vi "Add Event Reference to maps.vi"(7 "New Node Path":string, 8 "Event type":T1, 9 "Event VIs":refnum<vi>[](array[refnum]), 10 "Tree Map in":T2, 11 "map ref in":map{string, refnum<vi>}(c390)) -> (2 "Tree Map out":T2, 3 "map ref out":map{string, refnum<vi>}(c390))   [LabVIEW 2019, in "Panther Dashboard.lvlib"]
uses:
  Panther Dashboard.lvlib
  <vilib>/National Instruments/Tree Map/Tree Map Data.ctl
  Event types--enum.ctl
  <vilib>/National Instruments/Tree Map/Tree Map.lvlib
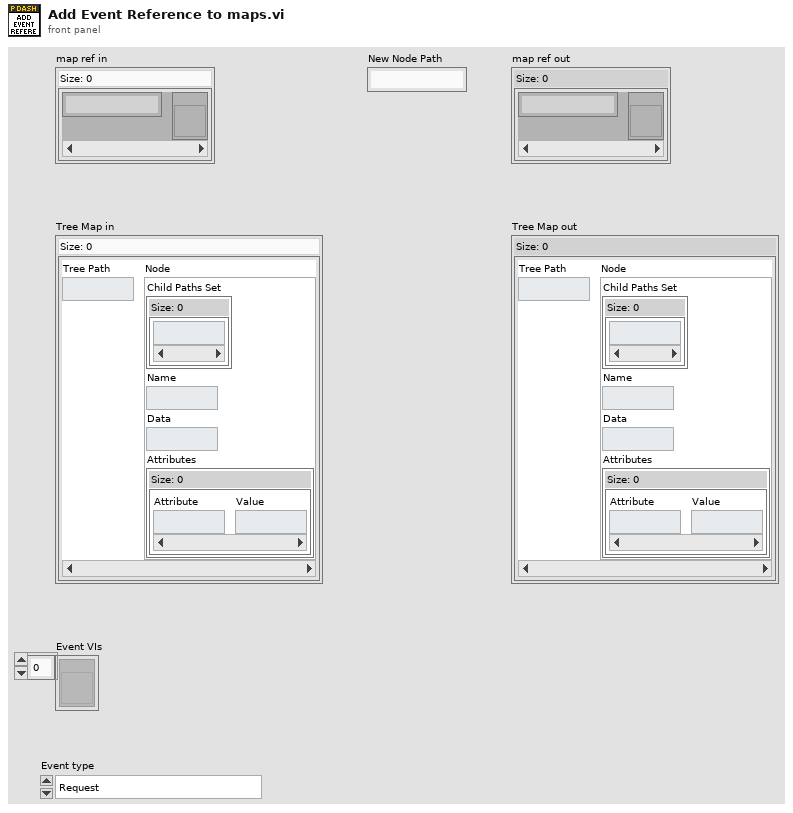
[diagram p1: front panel]
types:
  T1 = typedef "Panther Dashboard.lvlib/Event types--enum.ctl" = enum16{"Request", "Request and Wait for Reply", "Broadcast"}
  T2 = typedef "Tree Map.lvlib/Tree Map Data.ctl" = map{string, cluster{"Child Paths Set":set{string}, "Name":string, "Data":string, "Attributes":map{string, string}}}
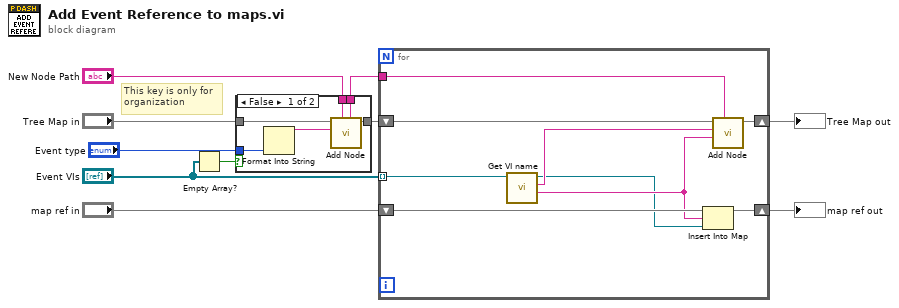
[diagram p0: block diagram]
diagram:
  # "This key is only for\norganization"
  n1 = Empty Array?(array="Event VIs") -> (empty?=w1:bool)
  n2 = case shown="False" w1 {
    tunnel: "New Node Path" -> [w15 w18]
    tunnel: [w14 w18] -> w6
    tunnel: "Tree Map in" -> [w13 w17]
    tunnel: [w12 w17] -> w4
    tunnel: "Event type" -> [w11 _]
    frame False {
      n3 = Format Into String(w11) -> (resulting string=w16:string)  [unwired: 3 in, 1 out]
      n4 = call <vilib>:"Add Node.vi"("Parent Path"=w15, "New Node Name"=w16, "Tree Map In"=w13) -> ("Tree Map Out"=w12:T2, "New Node Path"=w14:string)  [unwired: 6 in, 1 out]
    }
    frame True {
    }
  }
  n5 = for {
    tunnel: w6 -> [w27]
    shift-right: [w25] -> w10
    shift-left: w4 -> [w26]
    shift-right: [w23] -> w8
    shift-left: "map ref in" -> [w24]
    tunnel: "Event VIs" -> [w21] mode=indexing
    n6 = call "Get VI name.vi"("VI in"=w21) -> ("Full Vi Name"=w20:string, "Plain Name"=w22:string, "VI out"=w19:refnum<vi>)  [unwired: 8 in]
    n7 = Insert Into Map(map in=w24, key=w20, value=w19) -> (map out=w23:map{string, refnum<vi>})  [unwired: 2 out]
    n8 = call <vilib>:"Add Node.vi"("Parent Path"=w27, "Data"=w20, "New Node Name"=w22, "Tree Map In"=w26) -> ("Tree Map Out"=w25:T2)  [unwired: 5 in, 2 out]
  }
  "Tree Map out" <- w10
  "map ref out" <- w8
